vi "QT_FGGrab.vi"(0 "QT Ref In":T3, 2 "Compression Settings":T6 {"Dialogs" format="%.0b"; "Comp. Quality" format="%.0x"; "Codec" format="%.0x"}, 3 "Video Settings in":T5 {"Dialogs" format="%.0b"; "Color format" items=["Black & White (8 bits)", "RGB (24 bits)", "RGBx (32 bits)", "RGBA (32bits)", "RGB B&W (32 bits)", "HSI (24 bits)", "HSIx (32 bits)", "HSI B&W (32 bits)"]; "Brightness" format="%.2f"; "Contrast" format="%.2f"; "Sharpness" format="%.2f"; "Black Level" format="%.2f"; "White Level" format="%.2f"; "Saturation" format="%.2f"; "Hue" format="%.2f"}, 5 "error in (no error)":errorcluster, 8 "Private":T4) -> (9 "Info Out":T1, 14 "QT Ref Out":T3, 16 "Image/Movie Out":T2 {"Dialogs" format="%.0b"}, 19 "error out":errorcluster={"status"=TRUE, "code"=-43, "source"=""})   [LabVIEW 2024]
doc: "Retreive the most recent image from the given Frame grabber channel"
uses:
  <userlib>/ImageProcessing/QTLIB_2595_LV86/QT_Selector.ctl
  <userlib>/ImageProcessing/QTLIB_2595_LV86/QT_Compression.ctl
  <userlib>/ImageProcessing/QTLIB_2595_LV86/QT_Video.ctl
  <userlib>/ImageProcessing/QTLIB_2595_LV86/QT_Ref.ctl
  <userlib>/ImageProcessing/QTLIB_2595_LV86/QT_Private.ctl
  <userlib>/ImageProcessing/QTLIB_2595_LV86/QT_Image.ctl
  <userlib>/ImageProcessing/QTLIB_2595_LV86/QT_ErrInfo.ctl
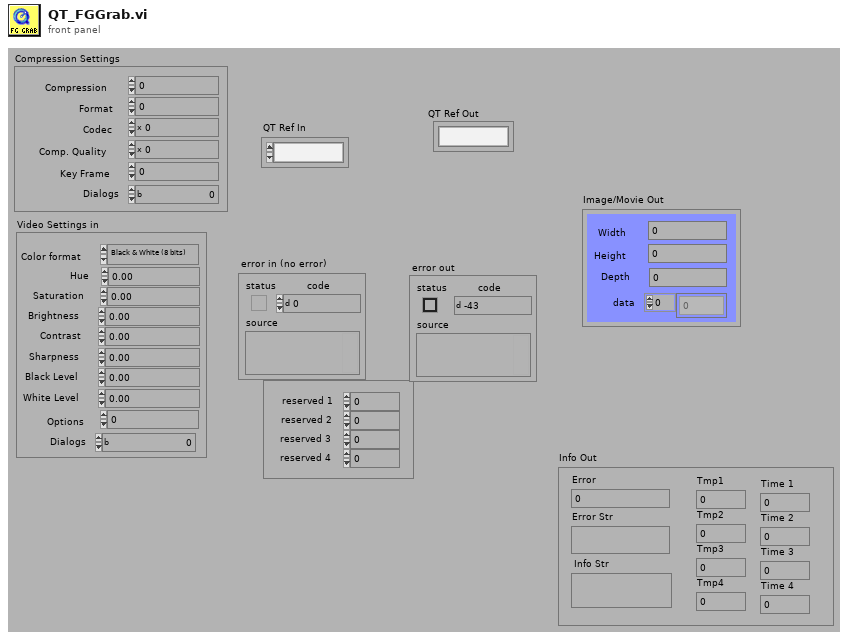
[diagram p1: front panel]
types:
  T1 = typedef "QT_ErrInfo.ctl" = cluster{"Error":i32, "Error Str":string, "Info Str":string, "Tmp1":i32, "Tmp2":i32, "Tmp3":i32, "Tmp4":i32, "Time 1":i32, "Time 2":i32, "Time 3":i32, "Time 4":i32}
  T2 = typedef "QT_Image.ctl" = cluster{"Width":i32, "Height":i32, "Depth":i32, "data":u8[], "Compressed data":u8[], "Color table":u32[], "Duration":i32, "Options":i32, "Timestamp":i32, "ID":i32, "Reserved":i32, "Dialogs":u32}
  T3 = typedef "QT_Ref.ctl" = refnum<k1>
  T4 = typedef "QT_Private.ctl" = cluster{"reserved 1":i32, "reserved 2":i32, "reserved 3":i32, "reserved 4":i32}
  T5 = typedef "QT_Video.ctl" = cluster{"Color format":u32, "Hue":dbl, "Saturation":dbl, "Brightness":dbl, "Contrast":dbl, "Sharpness":dbl, "Black Level":dbl, "White Level":dbl, "Options":i32, "Dialogs":u32}
  T6 = typedef "QT_Compression.ctl" = cluster{"Compression":i32, "Format":i32, "Codec":i32, "Comp. Quality":i32, "Key Frame":i32, "Dialogs":u32}
  T7 = typedef "QT_Selector.ctl" = enum32{"do nothing", "Get all Sources", "Get Source info", "Open Image", "Save Image to File", "Effect", "Close", "SG Grab", "Compress in Memory", "Decompress to Memory", "New Movie", "Open Movie", "Add Frame", "Get Frame", "Close Movie", "Get QT & CIN info", "SG init", "SG Close", "Open sound file", "Close sound file", "Read sound data", "Write sound data", "Import sound", "Export sound", "Add sound to movie", "Get sound from movie", "reserved", "reserved 1", "reserved 2"}
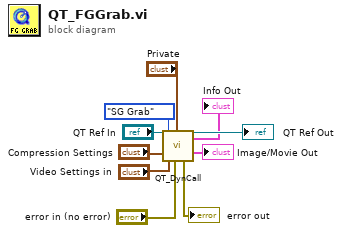
[diagram p0: block diagram]
diagram:
  n1 = call <userlib>:"QT_DynCall.vi"("QT Ref In"="QT Ref In", "Compression Settings"="Compression Settings", "error in (no error)"="error in (no error)", "Selector"=QT_Selector."SG Grab", "Video Settings in"="Video Settings in", "Private"="Private") -> ("Info Out"=→"Info Out":T1, "QT Ref Out"=→"QT Ref Out":T3, "Image/Movie Out"=→"Image/Movie Out":T2, "error out"=→"error out":errorcluster)  [unwired: 6 in, 12 out]
